vi "Write String.vi"(8 "error in (no error)":errorcluster, 10 "String":string, 11 "UDP in":refnum<class "UDP.lvclass">) -> (0 "error out":errorcluster, 3 "UDP out":refnum<class "UDP.lvclass">)   [LabVIEW 2018, in "UDP.lvclass"]
doc: "UDP.lvclass:Write String.vi\n\nThis is the template for the Write String VI for the UDP class.\n\nInstrument Communication Module Version 1.0\nJanuary, 2018 Original Code Consulting David Thomson\n www.originalcode.com i"
uses:
  UDP.lvclass
  UDP.lvclass/UDP.ctl
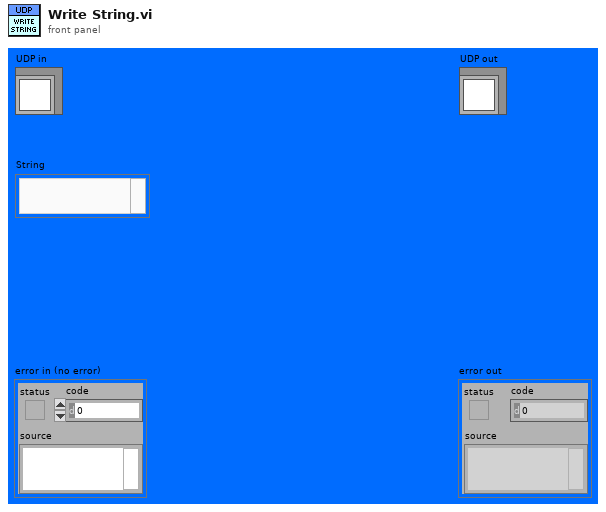
[diagram p1: front panel]
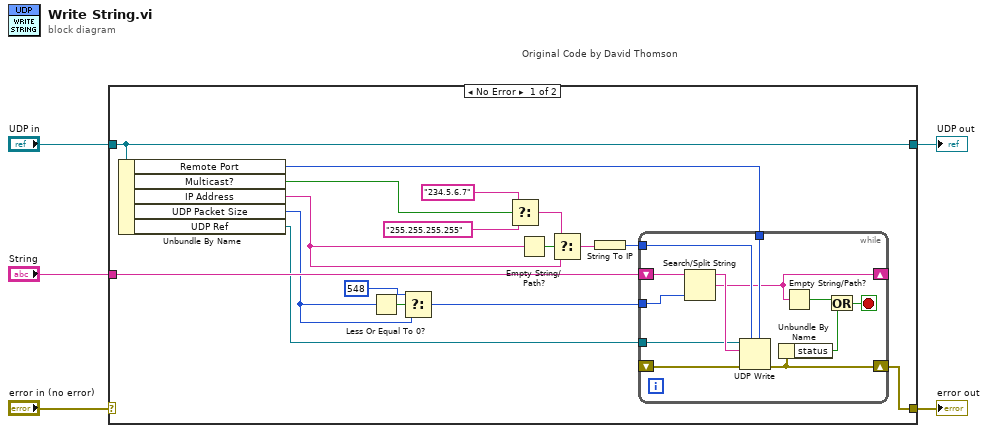
[diagram p0: block diagram]
diagram:
  n1 = case "Original Code by David Thomson" shown="No Error" "error in (no error)" {
    selector: "error in (no error)" -> [_ w36]
    tunnel: [w16 w36] -> w2
    tunnel: [w22 w35] -> w3
    tunnel: "UDP in" -> [w22 w35]
    tunnel: "String" -> [w18 _]
    frame No Error {
      n2 = Unbundle By Name(w22) -> ("Remote Port"=w15:u16, "Multicast?"=w7:bool, "IP Address"=w10:string, "UDP Packet Size"=w13:i32, "UDP Ref"=w17:refnum<k16>)
      n3 = Less Or Equal To 0?(x=w13) -> (x <= 0?=w19:bool)
      n4 = Select(t=548 ("max size (548)"), s=w19, f=w13) -> (s? t:f=w21:i32)
      n5 = Select(t="234.5.6.7", s=w7, f="255.255.255.255" ("t")) -> (s? t:f=w6:string)
      n6 = Empty String/Path?(string/path=w10) -> (empty?=w12:bool)
      n7 = Select(t=w6, s=w12, f=w10) -> (s? t:f=w11:string)
      n8 = String To IP(1:w11) -> (0:w14:u32)
      n9 = while {
        shift-right: [w28] -> _
        shift-left: w18 -> [w31]
        shift-right: [w26] -> w16
        shift-left: _ -> [w34]
        tunnel: w14 -> [w33]
        tunnel: w15 -> [w32]
        tunnel: w21 -> [w23]
        tunnel: w17 -> [w29]
        stop <- w24 stop-if-true
        n10 = Search/Split String(string=w31, offset (0)=w23) -> (substring before match=w30:string, match + rest of string=w28:string)  [unwired: 1 in, 1 out]
        n11 = UDP Write(address=w33, port or service name=w32, connection ID=w29, data in=w30, 8:w34) -> (error out=w26:errorcluster)  [unwired: 2 out]
        n12 = Unbundle By Name(w26) -> ("status"=w25:bool)
        n13 = Empty String/Path?(string/path=w28) -> (empty?=w27:bool)
        n14 = Or(x=w27, y=w25) -> (x .or. y?=w24:bool)
      }
    }
    frame Error {
    }
  }
  "error out" <- w2
  "UDP out" <- w3
